vi "Unibot.vi"() -> ()   [LabVIEW 2012]
doc: "Pendubot (Pendulum Robot) consists of a DC motor connected to a link physical rigid link (called here 'elbow\") which is connected to a second rigid link ('arm\") that has no actuation (free spinning link).\n\nThe control objective is to keep the free link in the vertical position while you can choose to balance the controller link (called here elbow) in the extended position (both links are up) or in the contracted position (elbow pointing down and free link up). In those operating points, a State Feedback Control is used to keep in Up-Up or Down-Up position.\n\nThis VI demonstrates how to use Linearization, design of LQR and pole placement controllers and use on swiching controller."
uses:
  <vilib>/addons/Control Design/_Model Construction/Model Typedefs.llb/CD State Space Model (MIMO).ctl
  <vilib>/addons/Control Design/_Model Construction/Model Typedefs.llb/CD General Elements.ctl
  <vilib>/Simulation/Scripting/Companion Diagram/SimConfigNode/SimParams.ctl
  <vilib>/Simulation/Scripting/Companion Diagram/SimConfigNode/_simSolvers.ctl
  <vilib>/Simulation/Implementation/Shared/SIMSCR Execution Mode.ctl
  <vilib>/Platform/TimedLoop/XDataNode/timing_clust.ctl
  <vilib>/Platform/TimedLoop/XDataNode/nitl_modes.ctl
  <vilib>/Platform/TimedLoop/XDataNode/wakeup.ctl
  <vilib>/Simulation/Param Hierarchy/Typedefs/SIMPH Param Control Actions.ctl
  <vilib>/Simulation/Scripting/Editor Utilities/SIM subVI tag data.ctl
  <vilib>/Simulation/Scripting/Editor Utilities/SIM subVI execution type.ctl
  <vilib>/Simulation/Implementation/Shared/NILVSim_ParamChanged.vi
  <vilib>/Simulation/Implementation/Shared/NILVSim_FinishedLate.vi
  <vilib>/Simulation/Utility/Implementation/SIM Halt.vi
  <vilib>/Simulation/SignalDisplay/Implementation/NILVSim Time Waveform.llb/SIM Time Waveform (scalar).vi
  <vilib>/Simulation/Implementation/Shared/SIM Fire Discrete SubVI.vi
  <vilib>/Simulation/Implementation/Shared/NILVSim_Manager.vi
  <vilib>/Simulation/Implementation/Shared/NILVSim_FinalizeModel.vi
  <vilib>/Simulation/Utility/Implementation/NILVSim Memory.llb/NILVSim Memory (core).vi
  <vilib>/Simulation/Implementation/Shared/SIM Is Init or Final Stage.vi
  <vilib>/Simulation/Implementation/Shared/SIM Fire Discrete SubVI (Core).vi
  <vilib>/addons/Control Design/_State Feedback Control/State Feedback Control.llb/State Feedback Control SubVis/cd_Discretized Linear Quadratic Regulator.vi
  <vilib>/Simulation/Implementation/Shared/SIM Unbundle Sim Info.vi
  <vilib>/Utility/error.llb/Clear Errors.vi
  <vilib>/Simulation/Implementation/Shared/NILVSim_GetModelError.vi
  <vilib>/Simulation/Implementation/Shared/SIM Bundle Sim Info.vi
  <vilib>/Simulation/Implementation/Shared/SIMSH Read Queue.vi
  <vilib>/Simulation/Implementation/Shared/NILVSim_Initialize.vi
  <vilib>/Simulation/Utility/Implementation/NILVSim Get Time and IsAcceptedStep.vi
  <vilib>/addons/Control Design/_Utility/Model Viewer.llb/Model Viewer SubVI/cd_Draw State-Space Equation (SS).vi
  <vilib>/addons/Control Design/_Model Conversions/Continuous and Discrete.llb/Continuous and Discrete SubVI/cd_Convert Continuous to Discrete (SS).vi
  <vilib>/addons/Control Design/_State Feedback Control/State Feedback Control.llb/CD State Regulator.vi
  <vilib>/addons/Control Design/_Model Reduction/Model Reduction.llb/Model Reduction SubVIs/cd_Remove I-O-S from SS Model.vi
  <vilib>/addons/Control Design/_Time Response Analysis/Time Response.llb/Time Response subVI/cd_Impulse Response (State-Space).vi
  <vilib>/addons/Control Design/_Time Response Analysis/Time Response.llb/Time Response subVI/cd_Parametric Time Response (SS with External Response).vi
  <vilib>/addons/Control Design/_Dynamic Analysis/Dynamic Analysis.llb/Dynamic Analysis subVI/cd_Stability (State-Space).vi
  <vilib>/addons/Control Design/_Dynamic Analysis/Dynamic Analysis.llb/Dynamic Analysis subVI/cd_Pole-Zero Map (State-Space).vi
  <vilib>/addons/Control Design/_Frequency Response Analysis/Frequency Response.llb/Frequency Response subVI/cd_Bode (State Space).vi
  Unibot - State Machine Controller.vi
  <vilib>/Simulation/Scripting/Companion Diagram/SimConfigNode/SimDog.xnode
  UniPend - NonLinear Model.vi
  <vilib>/Platform/TimedLoop/XDataNode/XDataNode.xnode
  <vilib>/Simulation/Implementation/XNodeFramework/SimXNode/SimX.xnode
  <vilib>/addons/Control Design/_State Feedback Control/NI_CD_State Feedback Control.lvlib
  <vilib>/addons/Control Design/_Utility/NI_CD_Model Viewer.lvlib
  <vilib>/addons/Control Design/_Model Reduction/NI_CD_Model Reduction.lvlib
  <vilib>/addons/Control Design/_Time Response Analysis/NI_CD_Time Response.lvlib
  <vilib>/addons/Control Design/_Utility/NI_LinSys_Polynomial Math.lvlib
  <vilib>/addons/Control Design/_Frequency Response Analysis/NI_CD_Frequency Response.lvlib
  <vilib>/addons/Control Design/_Model Conversions/NI_CD_Continuous and Discrete.lvlib
  <vilib>/addons/Control Design/_Dynamic Analysis/NI_CD_Dynamic Analysis.lvlib
  <vilib>/Platform/TimedLoop/XDataNode/XDNodeRunTimeDep.lvlib
  <vilib>/Simulation/Implementation/Shared/NI_SIM_Implementation.lvlib
  <vilib>/addons/Control Design/_Model Construction/NI_LinSys_Model Typedefs.lvlib
panel:
  in  "Parameters":T1={"Limit"=10.0, "Control Dead Band"=20.0, "Error Dead Band"=20.0}
  in  "dt (s) 2":dbl=10.0
  in  "y 2":dbl=100.0
  in  "Right":bool
  in  "Intensity":dbl(slide)=1.4000000000000001 scale=0.0..10.0
  in  "Left":bool
  in  "Mode":T2(ring)=enum."PID Balance"
  out "Control Effort":dbl(knob)=-0.004636384217224728 scale=-1000.0..1000.0
  out "Gain":dbl[][](array[numeric])=[[22309.46463411054, 3745.5012516070465]]
  out "State-Space Model":T3={"properties"={"Model name"="", "Input names"=["Torque (Tau)"], "Output names"=["alpha1"], "Input Delays"=[0.0], "Output Delays"=[0.0], "Sampling Time"=0.0, "Notes"=""}, "A"=[[0.0, 1.0], [-5.2843188746515235, 3.637978807091713e-12]], "B"=[[0.0], [0.049251038344664266]], "C"=[[0.9999999998191185, 0.0]], "D"=[[0.0]], "StateNames"=["/alpha", "/dalpha"], "Transport Delay"=[[0.0]]} {"Transport Delay" format="%.2f"; "D" format="%#.2g"; "C" format="%#.2g"; "B" format="%#.2g"; "A" format="%#.2g"; "properties"."Sampling Time" format="%#.6p"; "properties"."Output Delays" format="%.4f"; "properties"."Input Delays" format="%.4f"}
  in  "Tab Control":T5(tab)=enum."Simulation"
  in  "Start Open Loop":bool
  out "torque 2":waveform(dbl)(graph)={"t0"=timestamp(10.63 s since 1904-01-01), "dt"=1.0, "Y"=[0.0]}
  out "3D Picture Control 2":refnum<vi>(3d-picture)
  out "teta1 2":waveform(dbl)(graph)={"t0"=timestamp(10.63 s since 1904-01-01), "dt"=1.0, "Y"=[6.485760910217113]}
  in  "Initial Alpha (Angle)":dbl(knob) scale=-3.14..3.14
  in  "Iitial Beta":dbl(knob) scale=-3.14..3.14
  in  "Control Technique":T6(tab)=enum."Linear Quadratic Regulator"
  in  "Desired Pole Location":cdb[](array[numeric])=[-0.84+0.0i, 0.94+0.0i] format="%.2f"
  in  "Q":dbl[][](array[numeric])=[[10.0, 0.0], [0.0, 10.0]] format="%.2f"
  in  "R":dbl[][](array[numeric])=[[50.0]] format="%.2f"
  out "Optimal Gain \nDown-Up":dbl[](array[numeric])=[22309.46463411054, 3745.5012516070465] format="%.2f"
  out "Optimal Gain\nDown-Down":dbl[](array[numeric])=[-0.012293253837485524, 0.5949298178551672] format="%.2f"
  out "Optimal Gain \nUp-Up":dbl[](array[numeric])=[-16.081278889113918, -16.397482495141958, -3.1902773104017657, -2.0364914176335533] format="%.2f"
  in  "Type of Control":bool
  out "Linearized Equation for Operating Point":picture
  out "Poles locations":cdb[](array[numeric])=[0.9399999999999998+0.0i, -0.8400000000000057+0.0i] format="%.2f"
  out "Impulse Response":cluster{"time":dbl[], dbl[]}[](graph)
  out "Settling Time 1":dbl=0.7684673044317922
  out "Settling Time 2":dbl
  out "Bode Magnitude":cluster{"W":dbl[], "Magnitude":dbl[]}[](graph)=[{"W"=[0.01, 0.011768119524349986, 0.013848863713938732, 0.016297508346206444, 0.01917910261672489, 0.022570197196339205, 0.02656087782946687, 0.03125715849688237, 0.03678379771828634, 0.04328761281083059, 0.0509413801481638, 0.05994842503189412, 0.07054802310718646, 0.08302175681319748, 0.09770099572992257, 0.11497569953977363, 0.13530477745798075, 0.1592282793341093, 0.1873817422860385, 0.22051307399030468, 0.25950242113997374, 0.30538555088334174, 0.359381366380463, 0.42292428743895016, 0.4977023564332114, 0.5857020818056671, 0.6892612104349702, 0.8111308307896876, 0.9545484566618346, 1.123324032978028, 1.3219411484660297, 1.5556761439304727, 1.8307382802953693, 2.154434690031885, 2.5353644939701137, 2.983647240283341, 3.5111917342151338, 4.1320124001153395, 4.862601580065357, 5.722367659350222, 6.734150657750827, 7.92482898353918, 9.326033468832206, 10.974987654930569, 12.915496650148848, 15.199110829529348, 17.88649529057436, 21.049041445120217, 24.770763559917125, 29.150530628251786, 34.30469286314921, 40.37017258596558, 47.508101621028004, 55.90810182512228, 65.79332246575686, 77.42636826811278, 91.11627561154901, 107.22672220103243, 126.18568830660217, 148.49682622544665, 174.75284000076857, 205.65123083486537, 242.01282647943847, 284.8035868435805, 300.00997, 335.1602650938846, 394.420605943766, 464.15888336127847, 546.2277217684349, 600.0099399999999, 642.807311728433, 756.4633275546299, 890.2150854450398, 900.00991, 1047.6157527896662, 1200.0098799999998, 1232.8467394420677, 1450.8287784959416, 1707.352647470693, 2009.23300256505, 2364.4894126454105, 2782.559402207128, 3274.5491628777327, 3853.5285937105346, 4534.878508128588, 5336.699231206317, 6280.291441834261, 7390.722033525788, 8697.490026177846, 10235.310218990277, 12045.035402587839, 14174.741629268072, 16681.00537200061, 19630.406500402736, 23101.29700083163, 27185.882427329445, 31992.67137797388, 37649.35806792473, 44306.214575838865, 52140.082879996924, 61359.07273413182, 72208.09018385474, 84975.34359086455, 98500.00015, 98800.00012000001, 99100.00009, 99400.00006, 99700.00003, 100000.0], "Magnitude"=[-87.01146747990873, -87.01147184359166, -87.01147788678949, -87.01148625591792, -87.01149784618325, -87.01151389733282, -87.01153612625333, -87.01156691059501, -87.01160954305074, -87.01166858346822, -87.01175034641551, -87.01186357627103, -87.01202038189153, -87.0122375305317, -87.01253823883826, -87.01295465137542, -87.01353126965486, -87.01432969434875, -87.01543518006403, -87.0169656887314, -87.0190843811501, -87.02201682768194, -87.0260746737201, -87.03168809061307, -87.03945010168167, -87.0501768021031, -87.06498855211717, -87.0854182784335, -87.11355373863647, -87.15222030697419, -87.20520826694755, -87.27754164612905, -87.37577125120953, -87.50824928955507, -87.68530505659584, -87.91919557752686, -88.22367116962099, -88.6130126884884, -89.10051256058739, -89.69660002364057, -90.40707421261233, -91.23203129114998, -92.16590106016073, -93.1985880828671, -94.31729650050184, -95.50845661440073, -96.75930144066301, -98.05890668895975, -99.3987340021806, -100.7728295670367, -102.17784378622419, -103.61299904279437, -105.08007773374044, -106.5834471939854, -108.13008331017679, -109.72949862193079, -111.39342926652631, -113.13511156138652, -114.9680261786319, -116.90414682346554, -118.95198734154711, -121.11497719694357, -123.39072248913422, -125.77143016958223, -126.5523242318263, -128.2453191700142, -130.79849813737707, -133.4167423692146, -136.08680383874912, -137.64590812123635, -138.79715447420963, -141.53824993181252, -144.30247291414764, -144.48893545347337, -147.08390622349984, -149.4140110893679, -149.87804369308813, -152.68150323695994, -155.49177323528886, -158.30700284905274, -161.12583580732152, -163.94728228901099, -166.77062203888005, -169.59533207185785, -172.4210332286417, -175.24745092890822, -178.0743864868829, -180.90169621771028, -183.7292762556449, -186.55705154189098, -189.3849678469694, -192.21298599665909, -195.0410776955792, -197.86922250778207, -200.69740567456898, -203.52561653777036, -206.35384740070265, -209.18209270541263, -212.01034843843902, -214.83861170164982, -217.66688040231313, -220.4951530292832, -223.32342849137805, -225.8891556711362, -225.9419841430125, -225.99465244800965, -226.0471615543883, -226.0995124216554, -226.15170600066944]}]
  out "Bode Phase":cluster{"W":dbl[], "Magnitude":dbl[]}[](graph)=[{"W"=[0.01, 0.011768119524349986, 0.013848863713938732, 0.016297508346206444, 0.01917910261672489, 0.022570197196339205, 0.02656087782946687, 0.03125715849688237, 0.03678379771828634, 0.04328761281083059, 0.0509413801481638, 0.05994842503189412, 0.07054802310718646, 0.08302175681319748, 0.09770099572992257, 0.11497569953977363, 0.13530477745798075, 0.1592282793341093, 0.1873817422860385, 0.22051307399030468, 0.25950242113997374, 0.30538555088334174, 0.359381366380463, 0.42292428743895016, 0.4977023564332114, 0.5857020818056671, 0.6892612104349702, 0.8111308307896876, 0.9545484566618346, 1.123324032978028, 1.3219411484660297, 1.5556761439304727, 1.8307382802953693, 2.154434690031885, 2.5353644939701137, 2.983647240283341, 3.5111917342151338, 4.1320124001153395, 4.862601580065357, 5.722367659350222, 6.734150657750827, 7.92482898353918, 9.326033468832206, 10.974987654930569, 12.915496650148848, 15.199110829529348, 17.88649529057436, 21.049041445120217, 24.770763559917125, 29.150530628251786, 34.30469286314921, 40.37017258596558, 47.508101621028004, 55.90810182512228, 65.79332246575686, 77.42636826811278, 91.11627561154901, 107.22672220103243, 126.18568830660217, 148.49682622544665, 174.75284000076857, 205.65123083486537, 242.01282647943847, 284.8035868435805, 300.00997, 335.1602650938846, 394.420605943766, 464.15888336127847, 546.2277217684349, 600.0099399999999, 642.807311728433, 756.4633275546299, 890.2150854450398, 900.00991, 1047.6157527896662, 1200.0098799999998, 1232.8467394420677, 1450.8287784959416, 1707.352647470693, 2009.23300256505, 2364.4894126454105, 2782.559402207128, 3274.5491628777327, 3853.5285937105346, 4534.878508128588, 5336.699231206317, 6280.291441834261, 7390.722033525788, 8697.490026177846, 10235.310218990277, 12045.035402587839, 14174.741629268072, 16681.00537200061, 19630.406500402736, 23101.29700083163, 27185.882427329445, 31992.67137797388, 37649.35806792473, 44306.214575838865, 52140.082879996924, 61359.07273413182, 72208.09018385474, 84975.34359086455, 98500.00015, 98800.00012000001, 99100.00009, 99400.00006, 99700.00003, 100000.0], "Magnitude"=[-0.0957325014727103, -0.11265911554635381, -0.13257853436499598, -0.1560199071340693, -0.1836059338666657, -0.21606940055614318, -0.2542726343576648, -0.29923039279977, -0.35213679050208313, -0.4143969712468178, -0.48766435461092184, -0.5738844267937883, -0.675346206642382, -0.7947427014396589, -0.9352418727326224, -1.1005698577873966, -1.295108430144016, -1.524008918415144, -1.7933250080122158, -2.1101669761443644, -2.482879870704821, -2.921247795180363, -3.436725568931087, -4.04269721506798, -4.754757385513569, -5.591006035976078, -6.572337023441309, -7.722685834844279, -9.06917775701099, -10.642082502431007, -12.47443237523744, -14.601099734318252, -17.057066194027147, -19.874579903316913, -23.078948127751833, -26.682944307676696, -30.680320759424692, -35.039717046112266, -39.70109291482003, -44.57710059173264, -49.56085624008452, -54.53928516657689, -59.40866916490321, -64.08791804472746, -68.52625211050932, -72.70454059377381, -76.63178949464661, -80.33917324625472, -83.87367375908742, -87.29251827212312, -90.65877516686464, -94.03791023148787, -97.49481684028072, -101.09072822487364, -104.87944421337167, -108.90247257221742, -113.18307003599543, -117.71984132654075, -122.48144946104982, -127.40473644697603, -132.3984704598541, -137.35346182704149, -142.15723369697818, -146.70922791736373, -148.09711689314017, -150.9322404263626, -154.77763333808218, -158.22451072307, -161.27486875437887, -162.86074197453433, -163.94713716937358, -166.26993812166572, -168.27701325396112, -168.40146014596314, -170.00357187847067, -171.2540961150139, -171.48391997734473, -172.75008158340876, -173.83111677505204, -174.7528924750527, -175.53812696134912, -176.2065860280883, -176.77535218684918, -177.25911878067896, -177.67048112957852, -178.02020972933894, -178.31749845827528, -178.57018544422812, -178.78494689896428, -178.96746562448624, -179.12257653927935, -179.25439177793976, -179.36640787924097, -179.46159741289836, -179.54248717346022, -179.61122483076477, -179.66963569220584, -179.71927101388974, -179.76144910060603, -179.79729025975797, -179.82774652143706, -179.85362690411307, -179.87561889096327, -179.8926971442274, -179.89302296189786, -179.89334680691468, -179.89366869713896, -179.8939886502166, -179.89430668358193]}]
  out "Pole-Zero Map":cluster{dbl[], dbl[]}[](graph)=[{[-6.192885143661272, -178.27694061922173], [0.0, 0.0]}, {[], []}] caption="Closed Loop System Poles"
  out "Stability":T7(ring)
  out "Zeros":cdb[](array[numeric]) format="%.4f"
  out "Poles":cdb[](array[numeric])=[-6.192885143661272+0.0i, -178.27694061922173+0.0i] format="%.4f"
  out "3D Picture Control":refnum<vi>(3d-picture)
  out "teta1":waveform(dbl)(graph)={"t0"=timestamp(0 s since 1904-01-01), "dt"=1.0, "Y"=[0.0]}
  out "teta2":waveform(dbl)(graph)={"t0"=timestamp(0 s since 1904-01-01), "dt"=1.0, "Y"=[0.0]}
  out "torque":waveform(dbl)(graph)={"t0"=timestamp(0 s since 1904-01-01), "dt"=1.0, "Y"=[-0.004636384217224728]}
  in  "Halt?":bool
  out "Switching State":string="PID Balance"
  in  "Setpoint":dbl(knob) step=0.01 scale=-0.1..0.1
  in  "Control":bool=TRUE
  in  "Kill":bool
  in  "Enable":bool=TRUE
  in  "PID gains":T8={"proportional gain (Kc)"=10.0, "integral time (Ti, min)"=0.0, "derivative time (Td, min)"=1.0} {"derivative time (Td, min)" format="%.3f"; "integral time (Ti, min)" format="%.10f"; "proportional gain (Kc)" format="%.3f"}
  # "Disturbance"
  # "Unicycle Robot Design"
  # "cRIO 9024 RT Controller"
  # "RoboteQ Motor Controller"
  # "MicroStrain 3DM-GX3-45"
  # "3-Phase 12 V Hub Motor"
  # "Sideways Motion"
  # "Forward-Backward Motion"
  # "Closed-Loop Feedback State Variable System"
  # "IMU Sensor Reading"
  # "State Feedback Controller\nwith state machine"
  # "Swing Up?"
  # "Swing Down?"
  # "Initialize"
  # "Home?"
  # "Home?"
  # "Control Technique"
  # "Desired\nOperating\nPoint"
  # "Hub Motor"
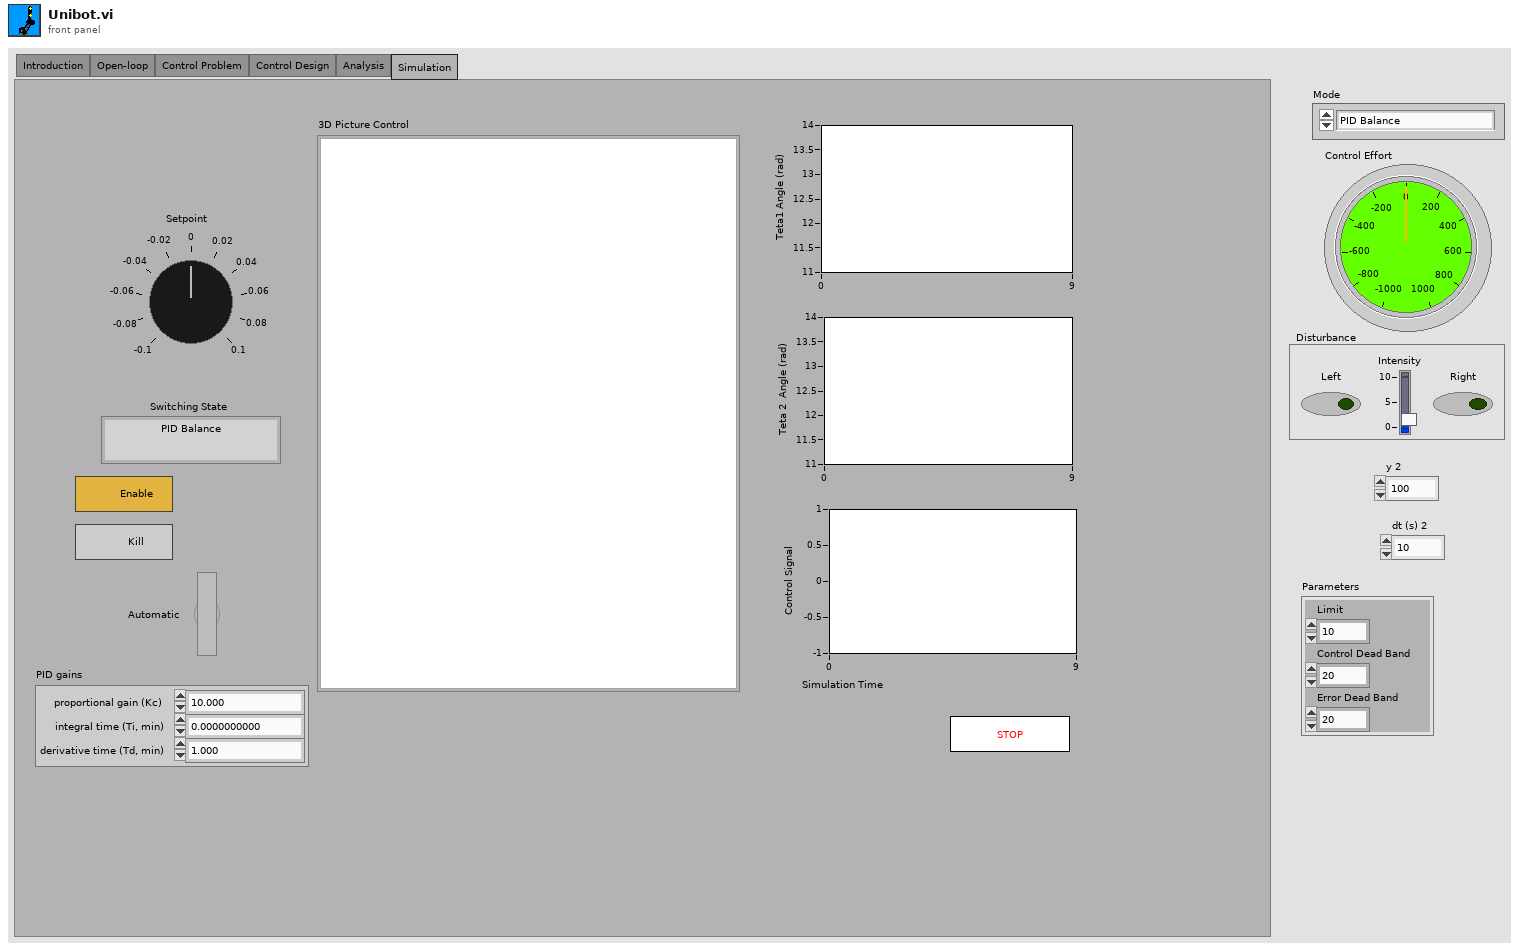
[diagram p1: front panel]
types:
  T1 = cluster{"Limit":dbl, "Control Dead Band":dbl, "Error Dead Band":dbl}
  T2 = enum16{"Idle", "Linear Balance", "Proportional Balance", "PID Balance", "Emergency"}
  T3 = typedef "NI_LinSys_Model Typedefs.lvlib/CD State Space Model (MIMO).ctl" = cluster{"properties":T4, "A":dbl[][], "B":dbl[][], "C":dbl[][], "D":dbl[][], "StateNames":string[], "Transport Delay":dbl[][]}
  T4 = typedef "NI_LinSys_Model Typedefs.lvlib/CD General Elements.ctl" = cluster{"Model name":string, "Input names":string[], "Output names":string[], "Input Delays":dbl[], "Output Delays":dbl[], "Sampling Time":dbl, "Notes":string}
  T5 = enum32{"Introduction", "Open-loop", "Control Problem", "Control Design", "Analysis", "Simulation"}
  T6 = enum32{"Pole Placement", "Linear Quadratic Regulator"}
  T7 = enum16{"stable", "marginally stable", "unstable", "undetermined"}
  T8 = cluster{"proportional gain (Kc)":dbl, "integral time (Ti, min)":dbl, "derivative time (Td, min)":dbl}
  T9 = typedef "SIMSCR Execution Mode.ctl" = enum16{"Simulate to Completion", "Single Time-Step Simulation (Fixed Step Only)"}
  T10 = typedef "XDNodeRunTimeDep.lvlib/timing_clust.ctl" = cluster{"Expected End [f-1]":u64, "Actual End [f-1]":u64, "Finished Late? [f-1]":bool, "Expected End [i-1]":u64, "Actual End [i-1]":u64, "Finished Late? [i-1]":bool, "Expected Start [i]":u64, "Actual Start [i]":u64, "Expected Start [f]":u64, "Actual Start [f]":u64, "Source Name":string, "Structure Name":string, "Period":i64, "Deadline":i64, "Offset":i64, "Start":i64, "Priority":i32, "Timeout":i32, "Mode":T11, "Wakeup Reason":T12, "Error":errorcluster, "Source Type":string, "Secondary Source Type":string, "Global End Time":u64, "Global Start Time":u64, "Frame Duration":u64, "Iteration Duration":u64, "Assigned CPU":i32, "I/O Scan Engine Mode":u32}
  T11 = typedef "XDNodeRunTimeDep.lvlib/nitl_modes.ctl" = enum32{"No Change", "Process missed periods, maintain original phase", "Discard missed periods, maintain original phase", "Process missed periods, ignore original phase", "Discard missed periods, ignore original phase"}
  T12 = typedef "XDNodeRunTimeDep.lvlib/wakeup.ctl" = enum32{"Normal", "Aborted", "Asynchronous wakeup", "Timing source error", "Timed loop error", "Timeout"}
  T13 = typedef "SIMPH Param Control Actions.ctl" = enum16{"get params", "set params"}
  T14 = typedef "SIM subVI tag data.ctl" = cluster{"period":dbl, "skew":dbl, "Simulation execution type":T15}
  T15 = typedef "SIM subVI execution type.ctl" = enum16{"Function call", "Discrete", "Continuous", "Initialization only", "Final step only"}
  T16 = cluster{"SIMSH Sim Time":dbl, "Build Array":cluster{"appended array":dbl[]}, "Unwrap Phase PtByPt.vi":cluster{"unwrapped phase":dbl}, "dalpha":cluster{"output":dbl}, "alpha":cluster{"output":dbl}, "Add 6":cluster{"x+y":dbl}, "Subtract 2":cluster{"x-y":dbl}, "Add 5":cluster{"x+y":dbl}, "Quotient & Remainder 2":cluster{"x-y*floor(x/y)":dbl}, "Multiply 8":cluster{"x*y":dbl}, "Formula Node":cluster{"d2alpha":dbl}}
  T17 = typedef "SimParams.ctl" = cluster{"Initial Time (s)":dbl, "Final Time (s)":dbl, "Step Size (s)":dbl, "ODE Solver":T18, "Minimum Step Size (s)":dbl, "Maximum Step Size (s)":dbl, "Relative Tolerance":dbl, "Absolute Tolerance":dbl, "Software Timing":bool, "Initial Step Size (s)":dbl, "Automatic Fixed Step Size?":bool, "Automatic Discrete Step Size?":bool, "Discrete Step Size (s)":dbl, "Calculate using Time Step":bool, "Solver Wired?":bool, "Prev.Frm.Expected End":u64, "Prev.Frm.Actual End":u64, "Prev.Frm.Finished Late?":bool, "Prev.Iter.Expected End":u64, "Prev.Iter.Actual End":u64, "Prev.Iter.Finished Late?":bool, "Expected Iteration Start":u64, "Actual Iteration Start":u64, "Expected Frame Start":u64, "Actual Frame Start":u64, "Source Name":string, "Name":string, "Period":i64, "Deadline":i64, "Offset":i64, "Start":i64, "Priority":i32, "Timeout":i32, "Processor":i32, "Mode":enum32{"No Change", "Process missed periods, maintain original phase", "Discard missed periods, maintain original phase", "Process missed periods, ignore original phase", "Discard missed periods, ignore original phase"}, "Wakeup reason":enum32{"Normal", "Aborted", "Asynchronous wakeup", "Timing source error", "Timed loop error", "Timeout"}, "Error":errorcluster, "Source Type":string, "Secondary Source Type":string, "Global End Time":u64, "Global Start Time":u64, "Full Solver Reset":bool, "Execution Mode":T9, "Nan/Inf Check":bool, "Custom Solver Library":string, "Solver Is Variable":bool, "custom solver name":string, "Signal Collection Decimation":u32}
  T18 = typedef "_simSolvers.ctl" = enum16{"Runge-Kutta 1 (Euler)", "Runge-Kutta 2", "Runge-Kutta 3", "Runge-Kutta 4", "Runge-Kutta 23 (variable)", "Runge-Kutta 45 (variable)", "BDF (variable)", "Adams-Moulton (variable)", "Rosenbrock (variable)", "Discrete States Only", "SDIRK 4 (variable)", "Radau 5 (variable)", "Radau 9 (variable)", "Radau 13 (variable)", "Radau [Variable Order] (variable)", "Gear's Method (variable)", "Linearizer", "State Query", "Trim Eval", "Custom Solver"}
  T19 = enum16{"System Included", "System Included with Noise", "Standalone"}
  T20 = enum8{"Enabled", "Disabled", "Disabled and Grayed Out"}
  T21 = typedef "NI_LinSys_Data Typedefs.lvlib/CD MIMO Time Response Data.ctl" = cluster{"Time":dbl[], "Outputs Data":dbl[][][], "States Data":dbl[][][], "plot type":T22}
  T22 = typedef "NI_LinSys_Data Typedefs.lvlib/CD Plot Types Enum.ctl" = enum16{"bode-magnitude", "bode-phase", "nichols", "nyquist", "singular values", "step", "impulse", "initial", "simulation", "nyquist with separation"}
  T23 = typedef "NI_LinSys_Data Typedefs.lvlib/CD Parametric Time Response Data.ctl" = cluster{"Rise Time (s)":dbl[][], "Peak Time (s)":dbl[][], "Settling Time (s)":dbl[][], "Overshoot (%)":dbl[][], "Steady-State Gain":dbl[][], "Peak Value":dbl[][]}
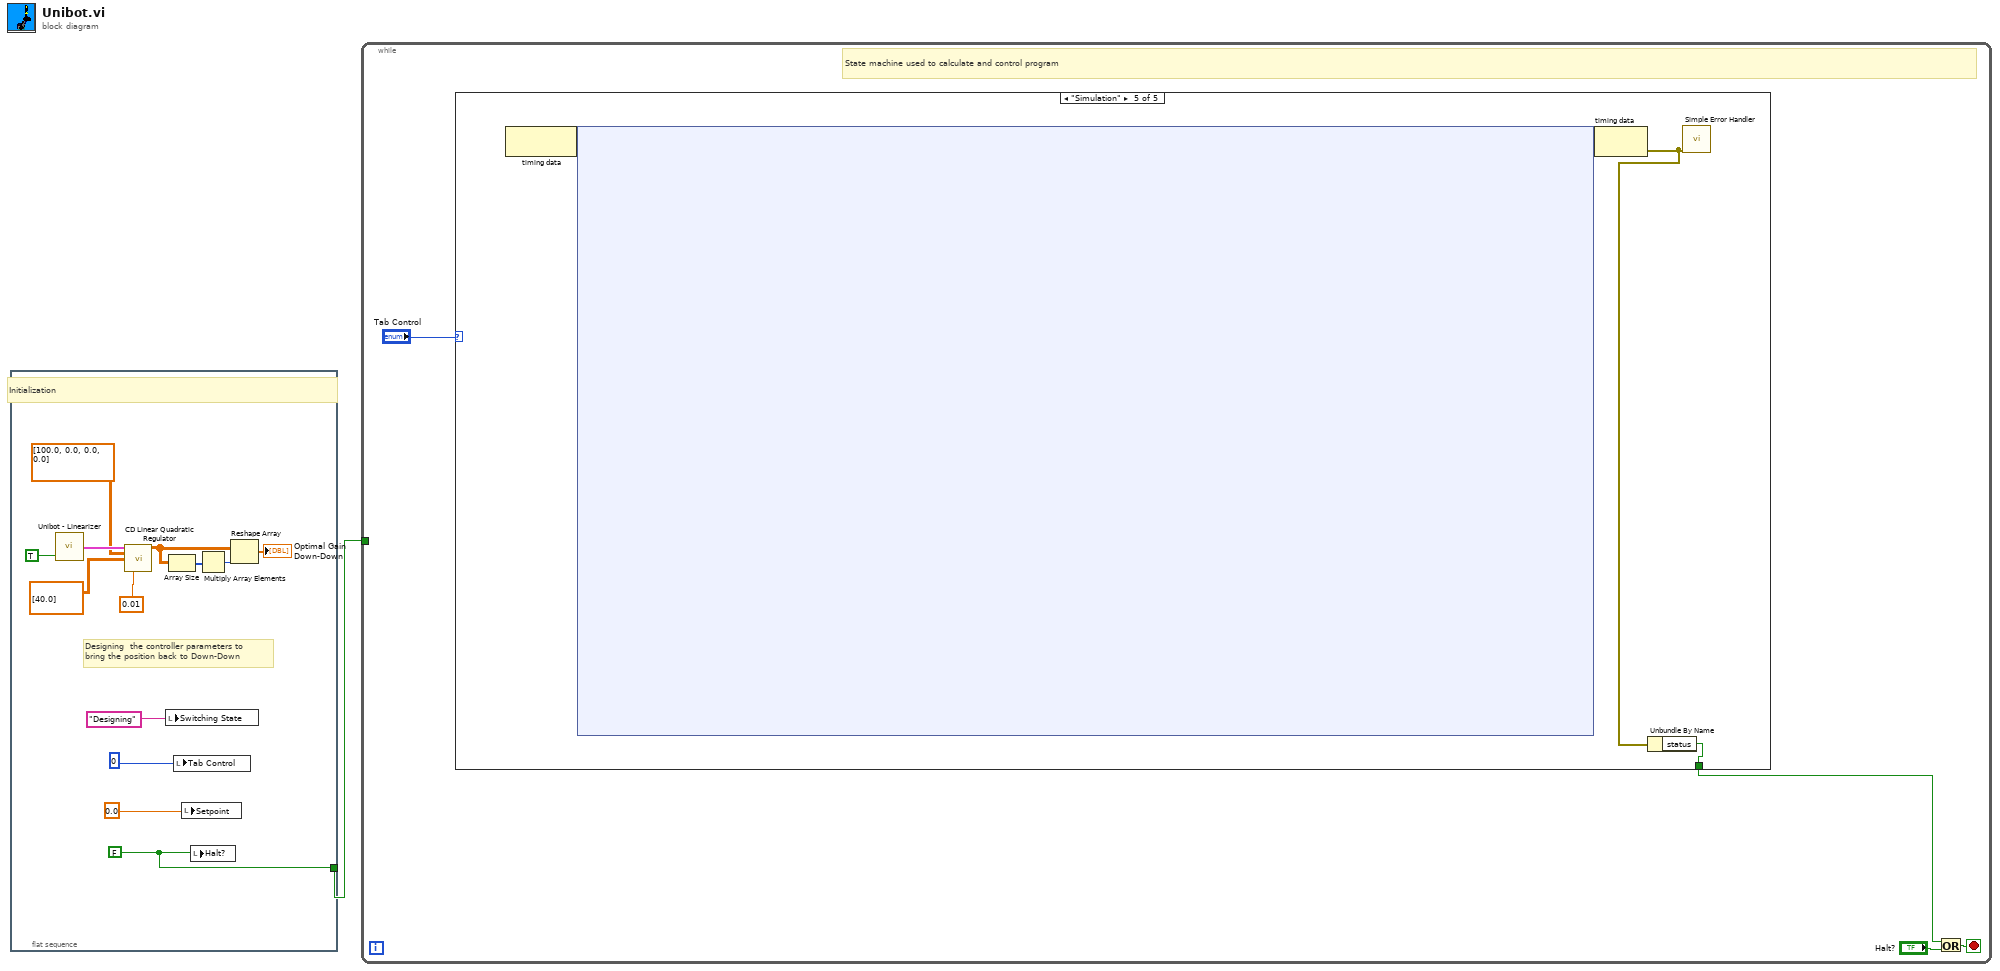
[diagram p0: block diagram]
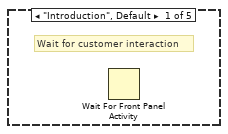
[diagram p2: hidden frame]
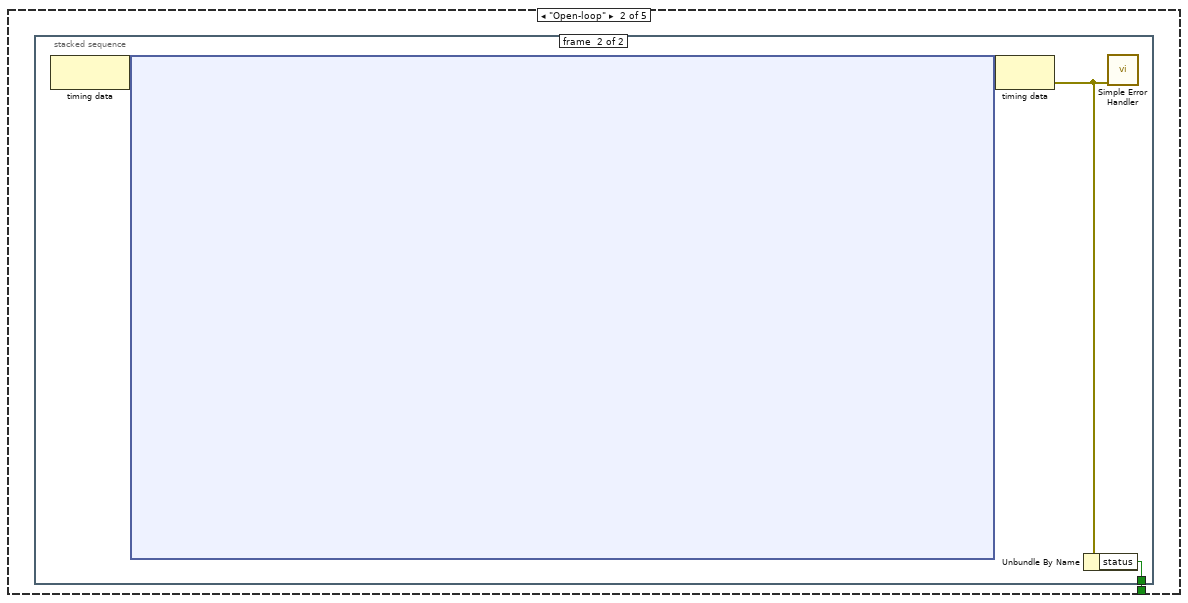
[diagram p3: hidden frame]
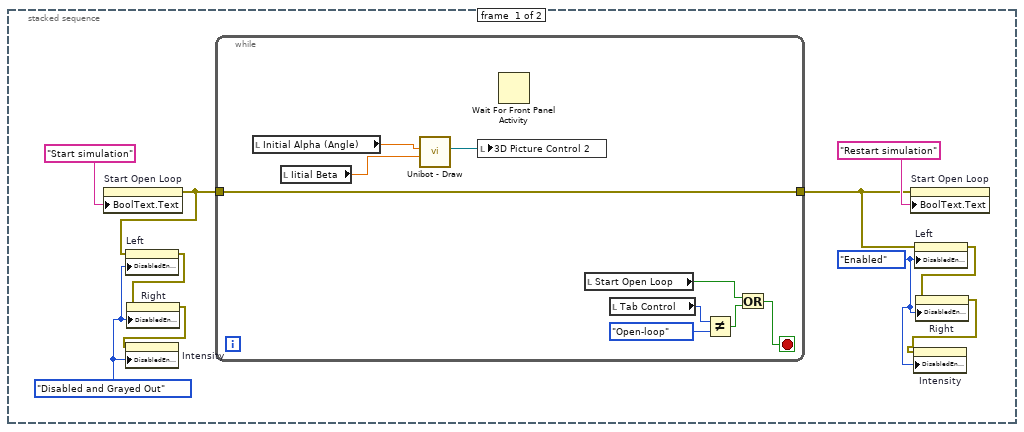
[diagram p4: hidden frame]
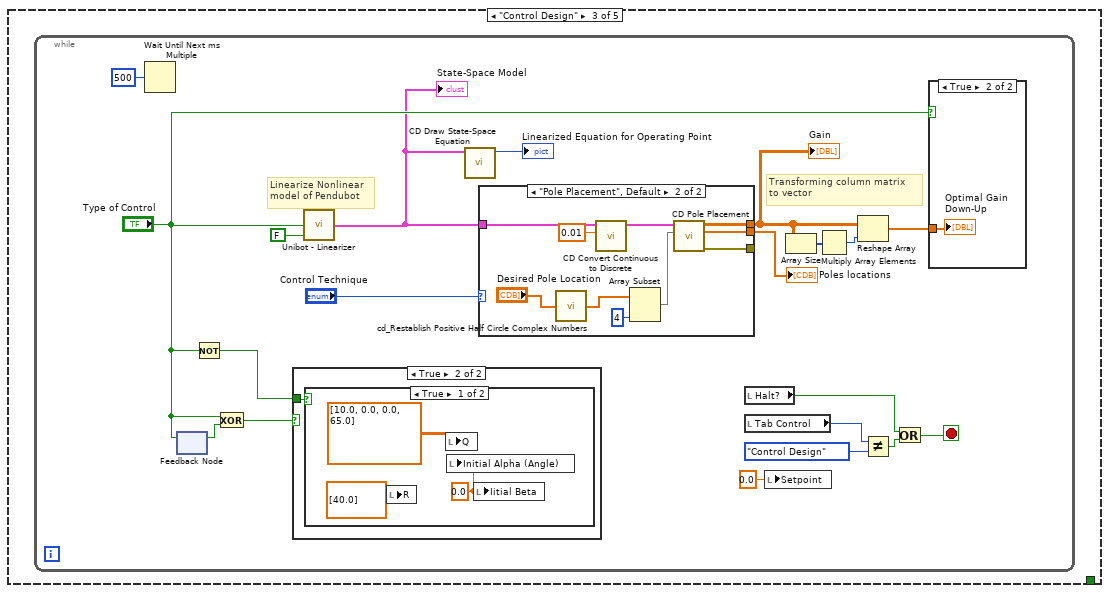
[diagram p5: hidden frame]
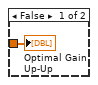
[diagram p6: hidden frame]
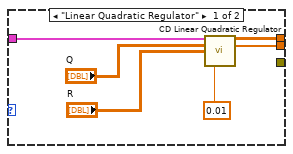
[diagram p7: hidden frame]
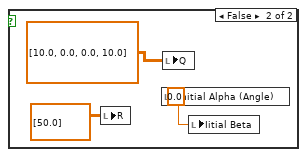
[diagram p9: hidden frame]
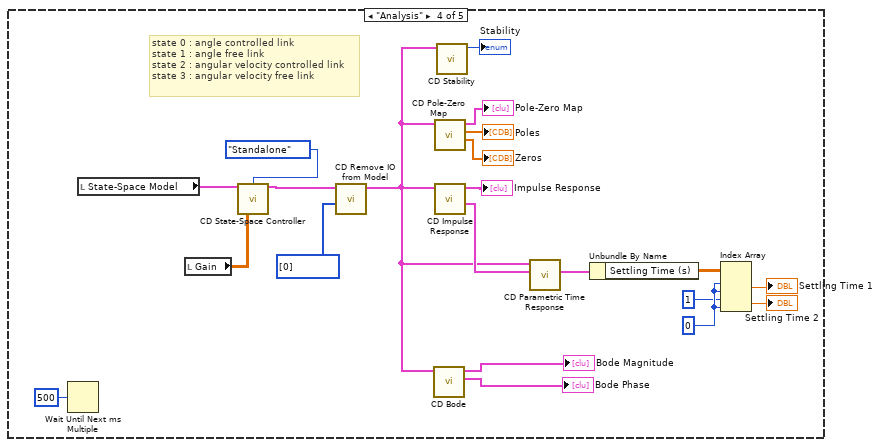
[diagram p10: hidden frame]
diagram:
  n1 = flat-sequence {
    tunnel: [w13] -> w1
    frame #0 {
      w13 = FALSE ("Halt?")
      # "Designing  the controller parameters to \nbring the position back to Down-Down"
      # "Initialization"
      n2 = call "Unibot - Linearizer.vi"("Up-Up"=TRUE ("Down-Down")) -> ("State-Space Model"=w11:T3)  [unwired: 1 in, 3 out]
      n3 = call-poly <vilib>:"CD Linear Quadratic Regulator.vi"("Continuous State-Space Model"=w11, "Q"=dbl[][] [[100.0, 0.0], [0.0, 0.0]], "R"=dbl[][] [[40.0]], "Sampling Time (s)"=0.01) -> ("Optimal Gain (K)"=w8:dbl[][])  [unwired: 2 in, 9 out]
      n4 = local write "Switching State"("Designing" ("Switching State")) -> ()
      n5 = Array Size(array=w8) -> (size(s)=w10:i32[])
      n6 = local write "Tab Control"(0 ("Setpoint")) -> ()
      n7 = local write "Setpoint"(0.0 ("Setpoint")) -> ()
      n8 = local write "Halt?"(w13) -> ()
      n9 = Multiply Array Elements(1:w10) -> (0:w9:i32)
      n10 = Reshape Array(w8, w9) -> (→"Optimal Gain\nDown-Down":dbl[])
    }
  }
  n11 = while {
    tunnel: w1 -> [_]
    stop <- w16 stop-if-true
    # "State machine used to calculate and control program"
    n12 = case shown="\"Simulation\"" "Tab Control" {
      tunnel: [_ w19 _ _ w483] -> w15
      frame "Introduction", Default {
        # "Wait for customer interaction"
        n13 = Wait For Front Panel Activity() -> ()  [unwired: 3 in, 1 out]
      }
      frame "Open-loop" {
        n14 = stacked-sequence {
          tunnel: [_ w39] -> w19
          frame #0 {
            w23 = T20."Disabled and Grayed Out" ("Disabled")
            w20 = T20."Enabled" ("Disabled")
            n15 = property on="Start Open Loop" class="Bool (strict)"("BoolText.Text"="Start simulation" ("Boolean Text.Text")) -> (error out=w26:errorcluster)  [unwired: 2 in, 1 out]
            n16 = property on="Left" class="Bool (strict)"(error in=w26, "DisabledEnum"=w23) -> (error out=w24:errorcluster)  [unwired: 1 in, 1 out]
            n17 = property on="Right" class="Bool (strict)"(error in=w24, "DisabledEnum"=w23) -> (error out=w22:errorcluster)  [unwired: 1 in, 1 out]
            n18 = property on="Intensity" class="Slide (strict)"(error in=w22, "DisabledEnum"=w23) -> ()  [unwired: 1 in, 2 out]
            n19 = while {
              tunnel: w26 -> [w30]
              tunnel: [w30] -> w27
              stop <- w31 stop-if-true
              n20 = local read "Initial Alpha (Angle)"() -> (w37:dbl)
              n21 = local read "Iitial Beta"() -> (w36:dbl)
              n22 = call "Unibot - Draw.vi"("Frame"=w36, "Motor"=w37) -> ("Rotated Scene Object"=w38:refnum<vi>)  [unwired: 9 in]
              n23 = local write "3D Picture Control 2"(w38) -> ()
              n24 = Wait For Front Panel Activity() -> ()  [unwired: 3 in, 1 out]
              n25 = local read "Start Open Loop"() -> (w32:bool)
              n26 = local read "Tab Control"() -> (w35:T5)
              n27 = Not Equal?(x=w35, y=T5."Open-loop") -> (x != y?=w33:bool)
              n28 = Or(x=w32, y=w33) -> (x .or. y?=w31:bool)
            }
            n29 = property on="Start Open Loop" class="Bool (strict)"(error in=w27, "BoolText.Text"="Restart simulation" ("Boolean Text.Text")) -> ()  [unwired: 1 in, 2 out]
            n30 = property on="Left" class="Bool (strict)"(error in=w27, "DisabledEnum"=w20) -> (error out=w25:errorcluster)  [unwired: 1 in, 1 out]
            n31 = property on="Right" class="Bool (strict)"(error in=w25, "DisabledEnum"=w20) -> (error out=w21:errorcluster)  [unwired: 1 in, 1 out]
            n32 = property on="Intensity" class="Slide (strict)"(error in=w21, "DisabledEnum"=w20) -> ()  [unwired: 1 in, 2 out]
          }
          frame #1 {
            n33 = node-c288() -> (w42:variant)  [unwired: 1 out]
            n34 = node-c254 ("Simulation Loop")(w42) -> (w41:variant)
            n35 = node-c288(w41) -> (w40:errorcluster)
            n36 = Unbundle By Name(w40) -> ("status"=w39:bool)
            n37 = call <vilib>:"Simple Error Handler.vi"("error in (no error)"=w40) -> ()  [unwired: 1 in, 8 out]
          }
        }
      }
      frame "Control Design" {
        n38 = while {
          stop <- w426 stop-if-true
          # "Linearize Nonlinear\nmodel of Pendubot"
          # "Transforming column matrix\nto vector"
          n39 = Wait Until Next ms Multiple(millisecond multiple=u32 500) -> ()  [unwired: 1 out]
          n40 = feedback-in #1("Type of Control") -> ()
          n41 = feedback #1() -> (w432:bool)  [unwired: 1 out]
          n42 = Not(x="Type of Control") -> (.not. x?=w430:bool)
          n43 = Exclusive Or(1:w432, 2:"Type of Control") -> (0:w431:bool)
          n44 = case shown="True" w431 {
            tunnel: w430 -> [_ w453]
            frame False {
            }
            frame True {
              n45 = case shown="True" w453 {
                frame True {
                  w454 = 0.0 ("initial teta2")
                  n46 = local write "R"(dbl[][] [[40.0]] ("R")) -> ()
                  n47 = local write "Q"(dbl[][] [[10.0, 0.0], [0.0, 65.0]] ("Q")) -> ()
                  n48 = local write "Initial Alpha (Angle)"(w454) -> ()
                  n49 = local write "Iitial Beta"(w454) -> ()
                }
                frame False {
                  w457 = 0.0 ("initial teta1")
                  n50 = local write "R"(dbl[][] [[50.0]] ("R")) -> ()
                  n51 = local write "Initial Alpha (Angle)"(w457) -> ()
                  n52 = local write "Q"(dbl[][] [[10.0, 0.0], [0.0, 10.0]] ("Q")) -> ()
                  n53 = local write "Iitial Beta"(w457) -> ()
                }
              }
            }
          }
          n54 = call "Unibot - Linearizer.vi"("Type of Control"="Type of Control", "Up-Up"=FALSE ("Down-Down")) -> ("State-Space Model"=w417:T3)  [unwired: 3 out]
          "State-Space Model" <- w417
          n55 = call-poly <vilib>:"CD Draw State-Space Equation.vi"("State-Space Model"=w417) -> ("Equation"=→"Linearized Equation for Operating Point":picture)  [unwired: 4 in, 6 out]
          n56 = case shown="\"Pole Placement\", Default" "Control Technique" {
            tunnel: [w442 w452] -> w418
            tunnel: w417 -> [w441 w448]
            tunnel: [w438 w451] -> w424
            tunnel: [_ w449] -> _
            frame "Linear Quadratic Regulator" {
              n57 = call-poly <vilib>:"CD Linear Quadratic Regulator.vi"("Continuous State-Space Model"=w441, "Q"="Q", "R"="R", "Sampling Time (s)"=0.01) -> ("Optimal Gain (K)"=w442:dbl[][], "Eigenvalues"=w438:cdb[])  [unwired: 2 in, 8 out]
            }
            frame "Pole Placement", Default {
              n58 = call <vilib>:"cd_Restablish Positive Half Circle Complex Numbers.vi"("Sorted Complex Numbers (Positive Only)"="Desired Pole Location") -> ("Complete Roots"=w445:cdb[])  [unwired: 8 out]
              n59 = call-poly <vilib>:"CD Convert Continuous to Discrete.vi"("Sampling Time (s)"=0.01, "Continuous State-Space Model"=w448) -> ("Discrete State-Space Model"=w447:T3)  [unwired: 7 in, 2 out]
              n60 = Array Subset(array=w445, length=4) -> (w443:cdb[])  [unwired: 1 in]
              n61 = call <vilib>:"CD Pole Placement.vi"("Poles"=w443, "State-Space Model"=w447) -> ("error out"=w449:errorcluster, "Actual Poles"=w451:cdb[], "Gain"=w452:dbl[][])  [unwired: 2 in, 5 out]
            }
          }
          "Poles locations" <- w424
          "Gain" <- w418
          n62 = local read "Halt?"() -> (w427:bool)
          n63 = local read "Tab Control"() -> (w425:T5)
          n64 = local write "Setpoint"(0.0 ("Gauge")) -> ()
          n65 = Array Size(array=w418) -> (size(s)=w434:i32[])
          n66 = Multiply Array Elements(1:w434) -> (0:w433:i32)
          n67 = Reshape Array(w418, w433) -> (w422:dbl[])
          n68 = Not Equal?(x=w425, y=T5."Control Design") -> (x != y?=w428:bool)
          n69 = Or(x=w427, y=w428) -> (x .or. y?=w426:bool)
          n70 = case shown="True" "Type of Control" {
            tunnel: w422 -> [w435 w436]
            frame False {
              "Optimal Gain \nUp-Up" <- w435
            }
            frame True {
              "Optimal Gain \nDown-Up" <- w436
            }
          }
        }
      }
      frame "Analysis" {
        w471 = 0 ("index (row)")
        # "state 0 : angle controlled link\nstate 1 : angle free link\nstate 2 : angular velocity controlled link\nstate 3 : angular velocity free link"
        n71 = Wait Until Next ms Multiple(millisecond multiple=u32 500) -> ()  [unwired: 1 out]
        n72 = local read "State-Space Model"() -> (w479:T3)
        n73 = local read "Gain"() -> (w477:dbl[][])
        n74 = call-poly <vilib>:"CD State-Space Controller.vi"("State-Space Model"=w479, "Configuration"=T19."Standalone", "Controller Gain (K)"=w477) -> ("Controller Model"=w476:T3)  [unwired: 11 in, 1 out]
        n75 = call-poly <vilib>:"CD Remove IO from Model.vi"("State-Space Model"=w476, "Outputs"=i32[] [0]) -> ("Reduced Model"=w464:T3)  [unwired: 7 in, 1 out]
        n76 = call-poly <vilib>:"CD Bode.vi"("State-Space Model"=w464) -> ("Bode Phase"=→"Bode Phase":cluster{"W":dbl[], "Magnitude":dbl[]}[], "Bode Magnitude"=→"Bode Magnitude":cluster{"W":dbl[], "Magnitude":dbl[]}[])  [unwired: 6 in, 3 out]
        n77 = call-poly <vilib>:"CD Pole-Zero Map.vi"("State-Space Model"=w464) -> ("Zeros"=→"Zeros":cdb[], "Poles"=→"Poles":cdb[], "Pole-Zero Map"=→"Pole-Zero Map":cluster{dbl[], dbl[]}[])  [unwired: 7 in, 1 out]
        n78 = call-poly <vilib>:"CD Impulse Response.vi"("State-Space Model"=w464) -> ("Impulse Response Data"=w474:T21, "Impulse Response Graph"=→"Impulse Response":cluster{"time":dbl[], dbl[]}[])  [unwired: 7 in, 2 out]
        n79 = call-poly <vilib>:"CD Stability.vi"("State-Space Model"=w464) -> ("Stability"=→"Stability":T7)  [unwired: 8 in, 2 out]
        n80 = call-poly <vilib>:"CD Parametric Time Response.vi"("Time Response Data"=w474, "State-Space Model"=w464) -> ("Time Response Parametric Data"=w473:T23)  [unwired: 8 in, 1 out]
        n81 = Unbundle By Name(w473) -> ("Settling Time (s)"=w465:dbl[][])
        n82 = Index Array(array=w465, index (row) #1=w471, index (col) #1=w471, index (row) #2=1 ("index (row)"), index (col) #2=w471) -> (element #1=→"Settling Time 1":dbl, element #2=→"Settling Time 2":dbl)
      }
      frame "Simulation" {
        n83 = node-c288() -> (w482:variant)  [unwired: 1 out]
        n84 = node-c254 ("Simulation Loop 2")(w482) -> (w481:variant)
        n85 = node-c288(w481) -> (w484:errorcluster)
        n86 = Unbundle By Name(w484) -> ("status"=w483:bool)
        n87 = call <vilib>:"Simple Error Handler.vi"("error in (no error)"=w484) -> ()  [unwired: 1 in, 8 out]
      }
    }
    n88 = Or(x=w15, y="Halt?") -> (x .or. y?=w16:bool)
  }
